vi "FP Analog Output.vi"() -> ()   [LabVIEW 2021]
uses:
  Analog Output/Analog Output/Analog Output.lvclass
panel:
  in  "Analog Output.lvlib:Analog Output.lvclass":refnum<class "Analog Output.lvclass">
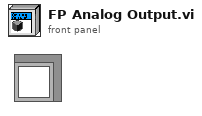
[diagram p1: front panel]
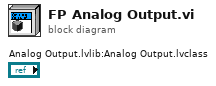
[diagram p0: block diagram]
diagram:
